vi "Write Saving.vi"(8 "error in (no error)":errorcluster, 10 "Saving":bool, 11 "Update Caller with File State in":refnum<class "Update Caller with File State.lvclass">) -> (0 "error out":errorcluster, 3 "Update Caller with File State out":refnum<class "Update Caller with File State.lvclass">)   [LabVIEW 2014, in "File Library.lvlib" / "Update Caller with File State.lvclass"]
uses:
  Update Caller with File State.lvclass
  Update Caller with File State.lvclass/Update Caller with File State.ctl
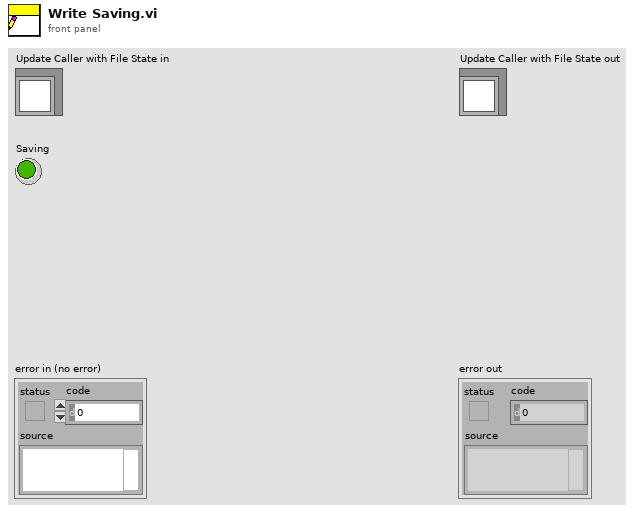
[diagram p1: front panel]
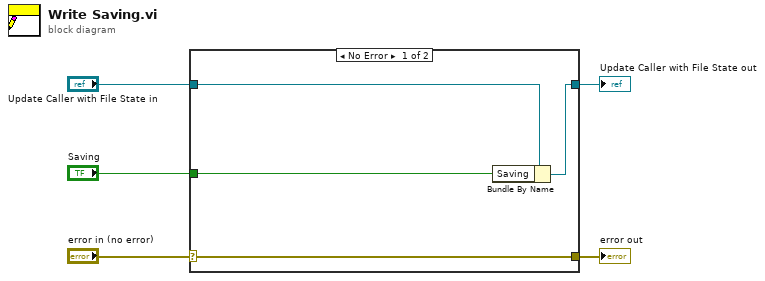
[diagram p0: block diagram]
diagram:
  n1 = case shown="No Error" "error in (no error)" {
    selector: "error in (no error)" -> [w9 w10]
    tunnel: [w9 w10] -> w4
    tunnel: [w7 w11] -> w2
    tunnel: "Update Caller with File State in" -> [w8 w11]
    tunnel: "Saving" -> [w6 _]
    frame No Error {
      n2 = Bundle By Name(cluster=w8, "Saving"=w6) -> (w7:refnum<class "Update Caller with File State.lvclass">)
    }
    frame Error {
    }
  }
  "error out" <- w4
  "Update Caller with File State out" <- w2
